vi "Write the VI.vi"(8 "error in (no error)":errorcluster, 11 "Paquetes Disonibles in":refnum<class "Paquetes Disonibles.lvclass">) -> (0 "error out":errorcluster, 3 "Paquetes Disonibles out":refnum<class "Paquetes Disonibles.lvclass">)   [LabVIEW 2021, in "Paquetes Disonibles.lvlib" / "Paquetes Disonibles.lvclass"]
uses:
  Paquetes Disonibles.lvclass
  Paquetes Disonibles.lvclass/Paquetes Disonibles.ctl
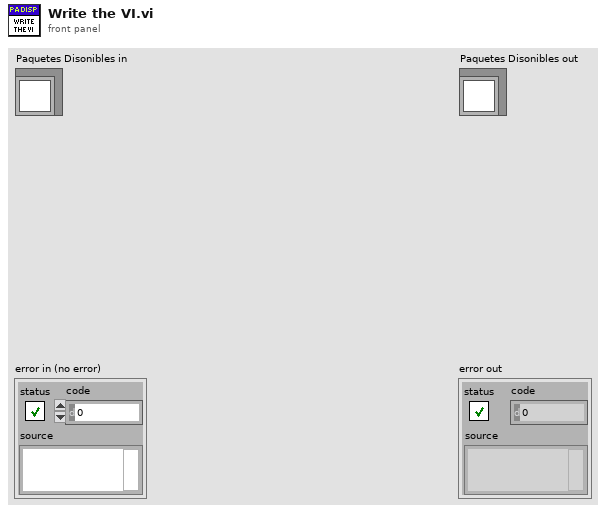
[diagram p1: front panel]
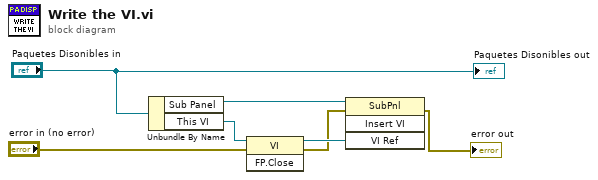
[diagram p0: block diagram]
diagram:
  n1 = Unbundle By Name("Paquetes Disonibles in") -> ("Sub Panel"=w7:refnum<vi>, "This VI"=w6:refnum<vi>)
  n2 = invoke class="VI" method="FP.Close"(reference=w6, error in="error in (no error)") -> (reference out=w5:refnum<vi>, error out=w4:errorcluster)  [unwired: 1 in, 1 out]
  n3 = invoke class="SubPnl" method="Insert VI"(reference=w7, error in=w4, "VI Ref"=w5) -> (error out=→"error out":errorcluster)  [unwired: 1 in, 3 out]
  "Paquetes Disonibles out" <- "Paquetes Disonibles in"
